vi "0_PatchCore_Train.vi"() -> ()   [LabVIEW 2020]
uses:
  PatchCore_AddOn/API/Controls/NN_Paths.ctl
  PatchCore_AddOn/API/Controls/PatchCore_Init_Custom_NN_CFG.ctl
  <vilib>/Ngene/Deep Learning Toolkit/Toolkit/NN_Data/API/NN_Dims(C,H,W).ctl
  <vilib>/Ngene/Deep Learning Toolkit/Toolkit/NN_Network/Controls/NN_Device.ctl
  PatchCore_AddOn/API/Controls/Coreset_Params.ctl
  PatchCore_AddOn/API/Controls/Random_Projection_Coreset.ctl
  PatchCore_AddOn/API/Controls/PCore_Device.ctl
  PatchCore_AddOn/API/Controls/Model_Saving_Params.ctl
  subVIs/Dataset_Reader/Controls/ImRead_PreProcessing_Options.ctl
  PatchCore_AddOn/Low_Level/Controls/Normalization_Type.ctl
  <vilib>/Analysis/baseanly.llb/Std Deviation and Variance.vi
  PatchCore_AddOn/API/NNPC_Generate_Embedding/NNPC_Generate_Embedding(Dataset).vi
  <vilib>/Ngene/Deep Learning Toolkit/Toolkit/Deep_Learning_Toolkit_by_Ngene.lvlib
panel:
  in  "PCore_Device":T1=enum."GPU(CuLab)"
  in  "Coreset_Params":T2={"Sampling_Ratio"=0.1, "Startd_idx"=3, "Random_Proj?"=TRUE, "Rnd. Proj. Params"={"Proj._Dim."=-1, "Epsilon"=0.9, "Seed"=42}}
  out "Coreset_Max_Distances":sgl[](graph)
  out "Generated_File_Paths":path[](array[path])=[path "D:/Ngene/Projects_SVN/DeepLTK/R_and_D/2024_02_01_Patchcore/LabVIEW/PatchCore_v5.0_cleaned_v1.1/Models/Patchcore_Models/__24_10_28__15_14_21/NNFE_WRN_50_2_L2L3_PS3_RP296.cfg", path "D:/Ngene/Projects_SVN/DeepLTK/R_and_D/2024_02_01_Patchcore/LabVIEW/PatchCore_v5.0_cleaned_v1.1/Models/Patchcore_Models/__24_10_28__15_14_21/NNFE_WRN_50_2_L2L3_PS3_RP296.bin", path "D:/Ngene/Projects_SVN/DeepLTK/R_and_D/2024_02_01_Patchcore/LabVIEW/PatchCore_v5.0_cleaned_v1.1/Models/Patchcore_Models/__24_10_28__15_14_21/PatchCore_Config.cfg", path "D:/Ngene/Projects_SVN/DeepLTK/R_and_D/2024_02_01_Patchcore/LabVIEW/PatchCore_v5.0_cleaned_v1.1/Models/Patchcore_Models/__24_10_28__15_14_21/MemBank_NNFE_WRN_50_2_L2L3_PS3_RP296_SR0.1_Size16.4k.bin"]
  in  "PatchCore_Dest_Folder_Path":path=path "D:/Ngene/Projects_SVN/DeepLTK/R_and_D/2024_02_01_Patchcore/LabVIEW/PatchCore_v5.0_cleaned_v1.1/Models/Patchcore_Models"
  in  "NNFE_Custom_CFG":T4={"Input3D_Custom_Dims"={"C"=3, "H"=224, "W"=224}, "mBatch"=1, "NN_Device"=enum."GPU"}
  in  "NNFE_Paths":T7={"CFG"=path "D:/working/Models/NN_Feature_Extractors/Patchcore_WRN_50_2_L2L3/Patchcore_WRN_50_2_L2L3.cfg", "BIN"=path "D:/working/Models/NN_Feature_Extractors/Patchcore_WRN_50_2_L2L3/Patchcore_WRN_50_2_L2L3.bin"}
  out "dT_Train_Total":dbl=24.56604519999999
  out "dT_Coreset":dbl=11.17188969999998
  out "dT_Gen_Embed":dbl=1.3900969999999973
  in  "Dataset_Path(Train)":path=path "D:/DNN/MVTec/bottle/train"
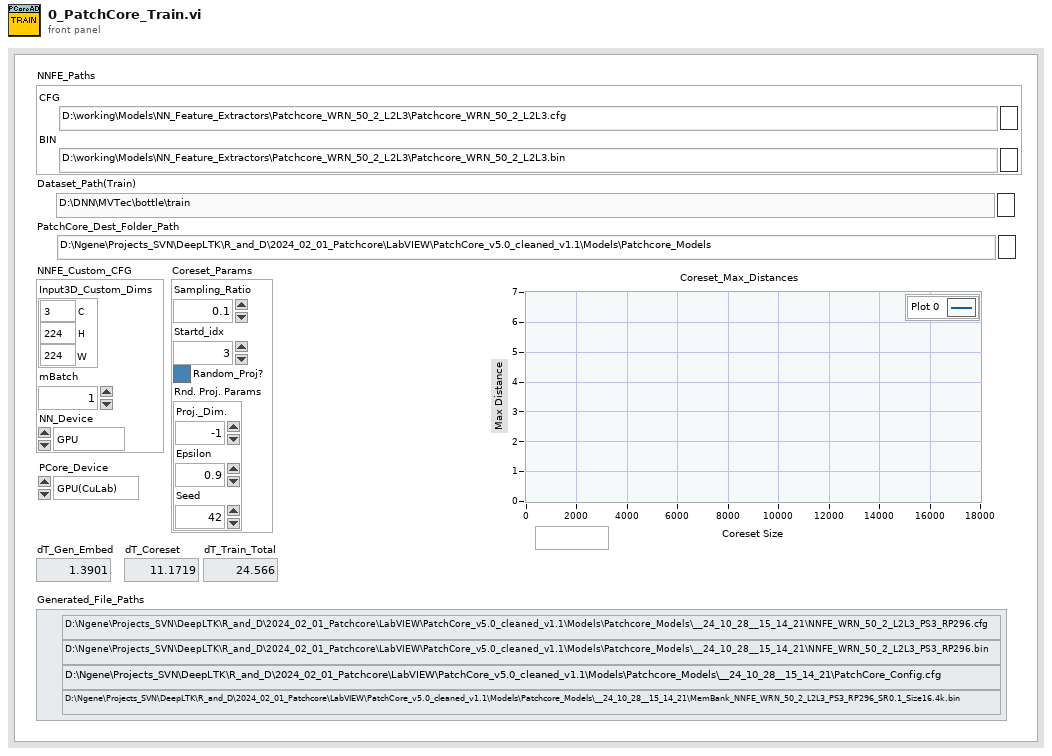
[diagram p1: front panel]
types:
  T1 = typedef "PCore_Device.ctl" = enum16{"CPU", "GPU(CuLab)"}
  T2 = typedef "Coreset_Params.ctl" = cluster{"Sampling_Ratio":sgl, "Startd_idx":i32, "Random_Proj?":bool, "Rnd. Proj. Params":T3}
  T3 = typedef "Random_Projection_Coreset.ctl" = cluster{"Proj._Dim.":i32, "Epsilon":sgl, "Seed":i32}
  T4 = typedef "PatchCore_Init_Custom_NN_CFG.ctl" = cluster{"Input3D_Custom_Dims":T5, "mBatch":i32, "NN_Device":T6}
  T5 = typedef "Deep_Learning_Toolkit_by_Ngene.lvlib/NN_Dims(C,H,W).ctl" = cluster{"C":i32, "H":i32, "W":i32}
  T6 = typedef "Deep_Learning_Toolkit_by_Ngene.lvlib/NN_Device.ctl" = enum16{"CPU", "GPU"}
  T7 = typedef "NN_Paths.ctl" = cluster{"CFG":path, "BIN":path}
  T8 = typedef "Model_Saving_Params.ctl" = cluster{"Save in Separate Folder?":bool}
  T9 = typedef "ImRead_PreProcessing_Options.ctl" = cluster{"Image Type":T10, "Normalization Type":T11, "Interpolation Type":u32}
  T10 = typedef "Image Type" = u32
  T11 = typedef "Normalization_Type.ctl" = enum16{"Standardize(DS_Stats)", "Standardize(Image_Stats)"}
  T12 = typedef "PatchCore_DS_Stats.ctl" = cluster{"means":T13, "vars":T13, "DS_Size":i32}
  T13 = typedef "Image_Stats_RGB.ctl" = cluster{"R":sgl, "G":sgl, "B":sgl}
  T14 = typedef "PatchCore_Instance.ctl" = cluster{"Dataset_Stats":T12, "NN":T15, "PCore_Device":T1, "PatchCore_Init_CFG":T30, "Coreset Params":T2, "MemBank_Data":T32}
  T15 = typedef "Deep_Learning_Toolkit_by_Ngene.lvlib/NN.ctl" = cluster{"Name":string, "No of Layers":i32, "mBatch":i32, "Layers":T16[], "Dimty":T17, "Dims_In":T5, "Dims_Out":T5, "Working_Dir":path, "Train?":bool, "Train_Params":T18, "LR_Update_Policy":T21, "Session Data":T23, "Ground_truth":T24, "NNg_hdls":T25, "NN_Device":T6, "GPU Id":i32, "Labels":string[], "Receptive Field":T26[], "Loss_Type":T27, "Loss_Cfg_Prms":variant, "NNG_WS":T28}
  T16 = typedef "Deep_Learning_Toolkit_by_Ngene.lvlib/NN_Layer_ref.ctl" = refnum<data-value>
  T17 = typedef "Deep_Learning_Toolkit_by_Ngene.lvlib/NN_In_Out_Dim-ty.ctl" = enum8{"In1D_Out1D", "In3D_Out1D", "In3D_Out3D", "In3D_OutBBox"}
  T18 = typedef "Deep_Learning_Toolkit_by_Ngene.lvlib/NN_Train_Params.ctl" = cluster{"Optimizer":T19, "Beta_1":sgl, "Beta_2":sgl, "Weight Decay(L1)":sgl, "Weight Decay(L2)":sgl, "Data_Sampling":T20}
  T19 = typedef "Deep_Learning_Toolkit_by_Ngene.lvlib/NN_Train_Optimizer.ctl" = enum16{"SGD", "Adam", "Adagrad", "Adadelta", "RMSProp", "Nesterov"}
  T20 = typedef "Deep_Learning_Toolkit_by_Ngene.lvlib/NN_Train_Data_Sampling.ctl" = enum16{"Random", "Sequential"}
  T21 = typedef "Deep_Learning_Toolkit_by_Ngene.lvlib/NN_LR_Policy_Cfg.ctl" = cluster{"Policy_Type":T22, "LR0":dbl, "k":sgl, "WarmUp_Policy":enum16{"Step", "Ramp"}, "WarmUp_Iter":i32, "WarmUp_Ratio":sgl}
  T22 = typedef "Deep_Learning_Toolkit_by_Ngene.lvlib/NN_LR_Policy_Type.ctl" = enum16{"Manual", "Step", "Exp", "1/t"}
  T23 = typedef "Deep_Learning_Toolkit_by_Ngene.lvlib/NN_Train_Session_Data.ctl" = cluster{"Epochs":sgl, "Tot_Iter":i32, "LR":sgl, "LR_iter":i32}
  T24 = typedef "Deep_Learning_Toolkit_by_Ngene.lvlib/NN_Ground_truth.ctl" = cluster{"Y":variant}
  T25 = typedef "Deep_Learning_Toolkit_by_Ngene.lvlib/nng_cuda_handles.ctl" = cluster{"cudnn":u64, "cublas":u64, "stream":u64, "curand":u64}
  T26 = typedef "Deep_Learning_Toolkit_by_Ngene.lvlib/NN_Dims(V,H).ctl" = cluster{"V":i32, "H":i32}
  T27 = typedef "Deep_Learning_Toolkit_by_Ngene.lvlib/NN_Loss_Type.ctl" = enum16{"None", "MSE", "CrossEntropy", "YOLO_v2", "YOLO_v4"}
  T28 = typedef "Deep_Learning_Toolkit_by_Ngene.lvlib/NNG_WS.ctl" = cluster{"NNG_WS_Mem":T29, "Max_WS_Size":i64}
  T29 = typedef "Deep_Learning_Toolkit_by_Ngene.lvlib/NNg_WS_Mem_DVR.ctl" = refnum<data-value>
  T30 = typedef "PatchCore_Init_CFG.ctl" = cluster{"BackBone":T31, "Out_Layers_Names":string[], "Patch_Size":u32}
  T31 = typedef "PatchCore_BackBone_Selector.ctl" = enum16{"WRN_50_2_L2L3"}
  T32 = typedef "MemBank_and_Norm_Variants.ctl" = cluster{"MemBank":variant, "MemBank Norm":variant}
  T33 = typedef "Deep_Learning_Toolkit_by_Ngene.lvlib/NN_DataSets_All(In3D_Out3D).ctl" = cluster{"Train":T34, "Validation":T34, "Test":T34}
  T34 = typedef "Deep_Learning_Toolkit_by_Ngene.lvlib/NN_DataSet(In3D_Out3D).ctl" = cluster{"Dataset_Size":i32, "Dims_In":T5, "Labels":string[], "File Paths":path[], "Outputs Ref.":T35, "Inputs Ref.":variant, "Dims_Out":T5}
  T35 = typedef "Deep_Learning_Toolkit_by_Ngene.lvlib/NN_Data_ref(4D_SGL).ctl" = refnum<data-value>
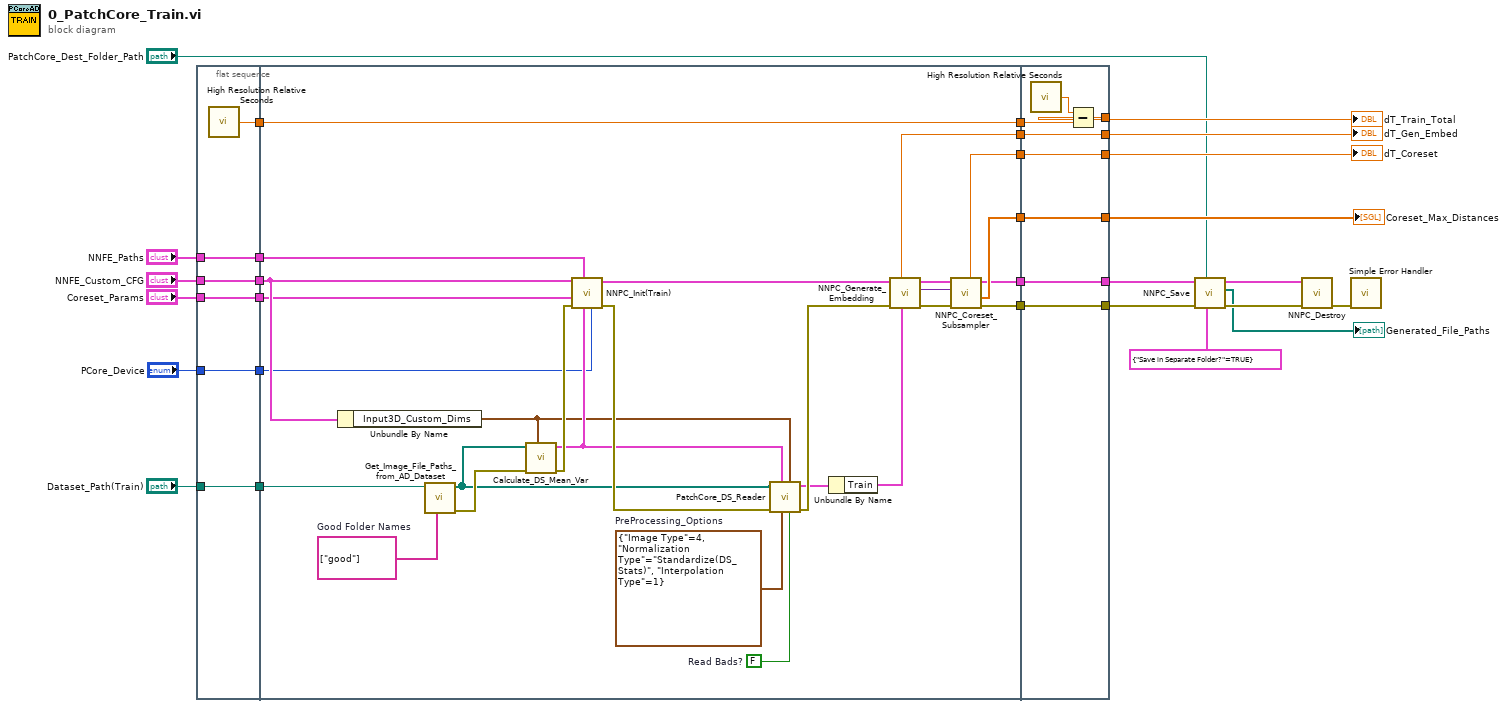
[diagram p0: block diagram]
diagram:
  n1 = flat-sequence {
    tunnel: [w35] -> w29
    tunnel: [w34] -> w24
    tunnel: "Dataset_Path(Train)" -> [w34]
    tunnel: [w33] -> w22
    tunnel: "Coreset_Params" -> [w33]
    tunnel: [w32] -> w21
    tunnel: "NNFE_Paths" -> [w32]
    tunnel: [w31] -> w19
    tunnel: "NNFE_Custom_CFG" -> [w31]
    tunnel: [w30] -> w2
    tunnel: "PCore_Device" -> [w30]
    tunnel: w29 -> [w62]
    tunnel: [w62] -> w28
    tunnel: [w61] -> w27
    tunnel: [w59] -> w25
    tunnel: w24 -> [w60]
    tunnel: w22 -> [w42]
    tunnel: w21 -> [w44]
    tunnel: w19 -> [w43]
    tunnel: [w55] -> w17
    tunnel: [w48] -> w10
    tunnel: [w47] -> w9
    tunnel: w2 -> [w38]
    tunnel: w28 -> [w69]
    tunnel: [w68] -> w26
    tunnel: [w67] -> w6
    tunnel: w27 -> [w67]
    tunnel: [w66] -> w13
    tunnel: w25 -> [w66]
    tunnel: [w65] -> w11
    tunnel: w17 -> [w65]
    tunnel: w10 -> [w64]
    tunnel: w9 -> [w63]
    tunnel: [w64] -> w7
    tunnel: [w63] -> w8
    frame #0 {
      n2 = call <vilib>:"High Resolution Relative Seconds.vi"() -> ("relative seconds"=w35:dbl)
    }
    frame #1 {
      w37 = T9 {"Image Type"=4, "Normalization Type"=enum."Standardize(DS_Stats)", "Interpolation Type"=1}  # PreProcessing_Options
      w39 = FALSE  # Read Bads?
      w54 = string[] ["good"]  # Good Folder Names
      n3 = Unbundle By Name(w43) -> ("Input3D_Custom_Dims"=w36:T5)
      n4 = call "Get_Image_File_Paths_from_AD_Dataset.vi"("Good Folder Names"=w54, "Dataset Folder"=w60) -> ("error out"=w58:errorcluster, "Good Dataset Files"=w40:path[])  [unwired: 7 in, 1 out]
      n5 = call "Calculate_DS_Mean_Var.vi"("Target Dims"=w36, "error in"=w58, "File Paths"=w40) -> ("error out"=w57:errorcluster, "Dataset_Stats"=w41:T12)  [unwired: 7 in]
      n6 = call "NNPC_Init(Train).vi"("PCore_Device"=w38, "Dataset_Stats"=w41, "NN_Paths"=w44, "error in (no error)"=w57, "Coreset_Params"=w42, "NNFE_Custom_CFG"=w43) -> ("error out"=w56:errorcluster, "PCore_Instance out"=w51:T14)  [unwired: 3 in, 1 out]
      n7 = call "PatchCore_DS_Reader.vi"("Read Bads?"=w39, "Input3D_Custom_Dims"=w36, "PreProcessing_Options"=w37, "Dataset_Stats"=w41, "error in"=w56, "Good Image File Paths"=w40) -> ("error out"=w53:errorcluster, "Dataset"=w46:T33)  [unwired: 4 in]
      n8 = Unbundle By Name(w46) -> ("Train"=w45:T34)
      n9 = call-poly "NNPC_Generate_Embedding.vi"("Dataset"=w45, "error in"=w53, "PCore_Instance in"=w51) -> ("error out"=w52:errorcluster, "Feature Embeddings"=w49:variant, "PCore_Instance out"=w50:T14, "dT_Embed"=w48:dbl)  [unwired: 4 in, 1 out]
      n10 = call "NNPC_Coreset_Subsampler.vi"("error in (no error)"=w52, "Features"=w49, "PCore_Instance in"=w50) -> ("error out"=w61:errorcluster, "max distances"=w59:sgl[], "PCore_Instance out"=w55:T14, "dT_Coreset"=w47:dbl)  [unwired: 4 in, 1 out]
    }
    frame #2 {
      n11 = call <vilib>:"High Resolution Relative Seconds.vi"() -> ("relative seconds"=w70:dbl)
      n12 = Subtract(x=w70, y=w69) -> (x-y=w68:dbl)
    }
  }
  n13 = call "NNPC_Save.vi"("Save_Options"=T8 {"Save in Separate Folder?"=TRUE} ("Save(T,T,T,T)"), "Dst Folder"="PatchCore_Dest_Folder_Path", "error in"=w6, "PCore_Instance in"=w11) -> ("error out"=w16:errorcluster, "Generated Files"=→"Generated_File_Paths":path[], "PCore_Instance out"=w4:T14)  [unwired: 5 in]
  n14 = call "NNPC_Destroy.vi"("error in"=w16, "PCore_Instance in"=w4) -> ("error out"=w15:errorcluster)  [unwired: 9 in]
  n15 = call <vilib>:"Simple Error Handler.vi"("error in (no error)"=w15) -> ()  [unwired: 4 in, 5 out]
  "dT_Train_Total" <- w26
  "Coreset_Max_Distances" <- w13
  "dT_Gen_Embed" <- w7
  "dT_Coreset" <- w8
